vi "Write Data.vi"(8 "error in (no error)":errorcluster, 10 "Data":dbl[](array[numeric]), 11 "RMS in":refnum<class "RMS.lvclass">) -> (0 "error out":errorcluster, 3 "RMS out":refnum<class "RMS.lvclass">)   [LabVIEW 2015]
uses:
  RMS.lvclass
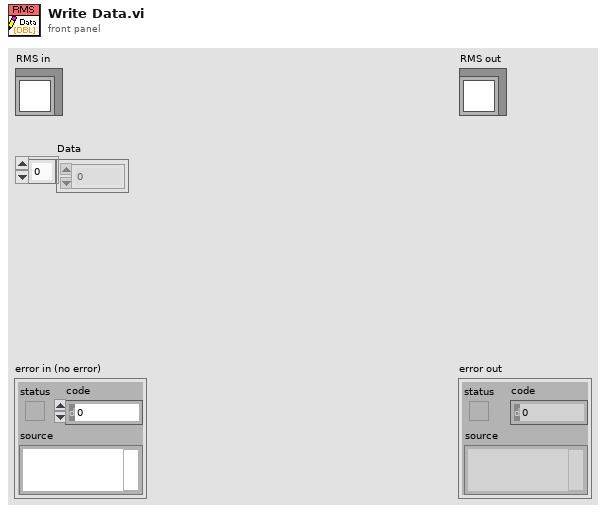
[diagram p1: front panel]
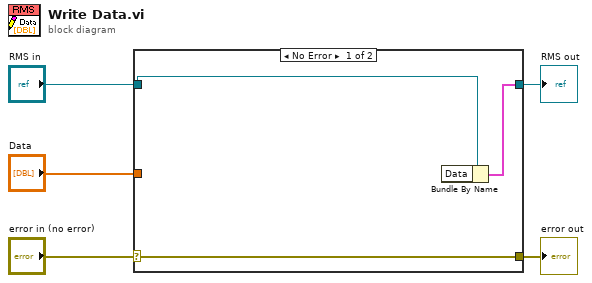
[diagram p0: block diagram]
diagram:
  n1 = case shown="No Error" "error in (no error)" {
    selector: "error in (no error)" -> [w8 w9]
    tunnel: [w8 w9] -> w4
    tunnel: [w6 w10] -> w2
    tunnel: "RMS in" -> [w7 w10]
    tunnel: "Data" -> [_ _]
    frame No Error {
      n2 = Bundle By Name(cluster=w7) -> (w6:cluster{})  [unwired: 1 in]
    }
    frame Error {
    }
  }
  "error out" <- w4
  "RMS out" <- w2
